vi "Apply Manipulation.vi"(8 "error in (no error)":errorcluster, 10 "Data in":dbl[][](array[numeric]), 11 "Desaccade Manipulator in":refnum<class "Desaccade Manipulator.lvclass">) -> (0 "error out":errorcluster, 2 "Data out":dbl[][](array[numeric]), 3 "Desaccade Manipulator out":refnum<class "Desaccade Manipulator.lvclass">)   [LabVIEW 2016, in "Desaccade Manipulator.lvclass"]
uses:
  Desaccade Manipulator.lvclass
  Desaccade Manipulator.lvclass/Desaccade Manipulator.ctl
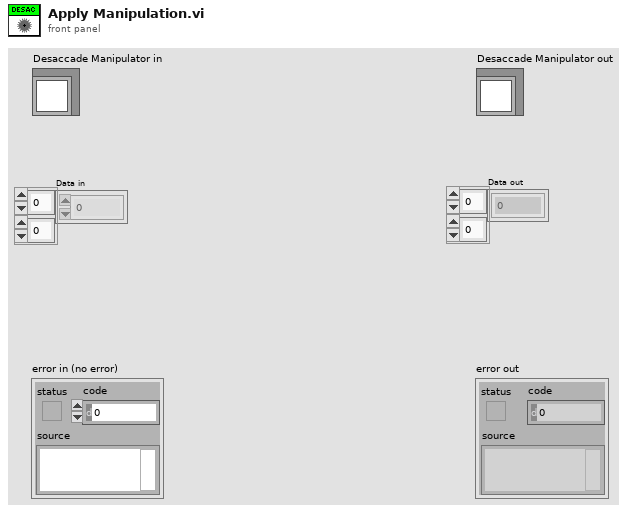
[diagram p1: front panel]
types:
  T1 = typedef "Typedef - Desaccading Parameter.ctl" = cluster{"Threshold 1 [Acc]":dbl, "Threshold 2 [% of TH1]":i32, "tolerance":dbl, "Search WD ":dbl, " always use TH2":bool, "SD for Outliers":dbl, "Max time [ms]":dbl, "Min time [ms]":dbl, "Velocity Threshold":dbl}
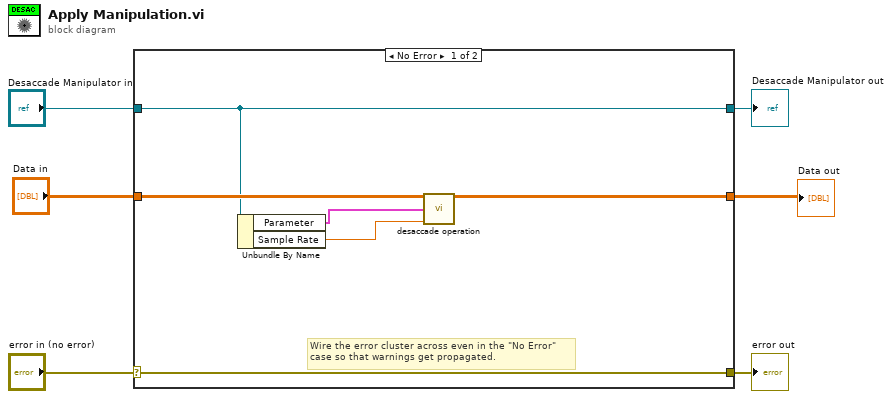
[diagram p0: block diagram]
diagram:
  n1 = case shown="No Error" "error in (no error)" {
    selector: "error in (no error)" -> [w12 w15]
    tunnel: [w12 w15] -> w5
    tunnel: [w9 w14] -> w3
    tunnel: "Desaccade Manipulator in" -> [w9 w14]
    tunnel: "Data in" -> [w11 w13]
    tunnel: [w10 w13] -> w1
    frame No Error {
      # "Wire the error cluster across even in the \"No Error\"\ncase so that warnings get propagated."
      n2 = Unbundle By Name(w9) -> ("Parameter"=w8:T1, "Sample Rate"=w7:dbl)
      n3 = call "desaccade operation.vi"("Data not diff"=w11, "Parameter"=w8, "Sample Rate"=w7) -> ("Desaccaded"=w10:dbl[][])  [unwired: 12 in]
    }
    frame Error {
    }
  }
  "error out" <- w5
  "Desaccade Manipulator out" <- w3
  "Data out" <- w1
